vi "PH_Beckhoff_PP_PU.ProcPeriodic.vi"(0 "i ref in":refnum<vi>, 3 "ms timeout (10000)":i32=10000, 5 "error in (no error)":errorcluster) -> (14 "i ref out":refnum<vi>, 17 "timed out":bool, 19 "error out":errorcluster)   [LabVIEW 2014, in "PH_Beckhoff_PP_PU.lvlib"]
doc: "This method serves to periodically do things like reading values from the HW. Methods that should be executed periodically should be called from THIS methode. Add code here."
uses:
  PH_Beckhoff_PP_PU.lvlib
  PH_Beckhoff/PH_Beckhoff.lvlib
  non_GPL/instr.lib/Beckhoff/Beckhoff - Driver np.lvlib
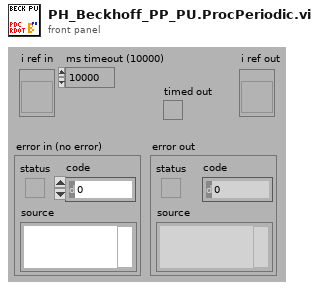
[diagram p1: front panel]
types:
  T1 = typedef "PH_Beckhoff_PP_PU.lvlib/PH_Beckhoff_PP_PU.i attribute.ctl" = cluster{"HV Meas":cluster{"Input GUI Ref":refnum<vi>, "Voltage Service ID":i32, "Voltage [V]":dbl, "Quality":bool, "# in Data":i32}[], "Trigger":cluster{"Status":cluster{"GUI Ref":refnum<vi>, "Status Service ID":i32, "Status":T2}, "last shot:":cluster{"GUI Ref":refnum<vi>, "Service ID":i32, "Time":string}, "DIs":cluster{"triggered":cluster{"GUI Ref":refnum<vi>, "# in Data":i32}, "fired":cluster{"GUI Ref":refnum<vi>, "# in Data":i32}}, "GUI Ref Indicator":refnum<vi>}[], "RR":cluster{"Status":cluster{"GUI Ref":refnum<vi>, "Status Service ID":i32, "Status":T2}, "DIs":cluster{"closed":cluster{"GUI Ref":refnum<vi>, "# in Data":i32}, "open":cluster{"GUI Ref":refnum<vi>, "# in Data":i32}}, "Close":cluster{"GUI Ref":refnum<vi>, "# in Data":i32}, "GUI Ref Indicator":refnum<vi>}[], "Igni":cluster{"Status":cluster{"GUI Ref":refnum<vi>, "Status Service ID":i32, "Status":T2}, "DIs":cluster{"heating on":cluster{"GUI Ref":refnum<vi>, "# in Data":i32}, "water on":cluster{"GUI Ref":refnum<vi>, "# in Data":i32}}, "Device on":cluster{"GUI Ref":refnum<vi>, "# in Data":i32}, "GUI Ref Indicator":refnum<vi>}[], "PSU":cluster{"Status":cluster{"GUI Ref":refnum<vi>, "Status Service ID":i32, "Status":T2}, "Limit Service ID":i32, "DIs":cluster{"inhibit":cluster{"GUI Ref":refnum<vi>, "# in Data":i32}, "end of charge":cluster{"GUI Ref":refnum<vi>, "# in Data":i32}, "HV on":cluster{"GUI Ref":refnum<vi>, "# in Data":i32}, "overtemp":cluster{"GUI Ref":refnum<vi>, "# in Data":i32}, "interlock":cluster{"GUI Ref":refnum<vi>, "# in Data":i32}, "load fault":cluster{"GUI Ref":refnum<vi>, "# in Data":i32}, "sum fault":cluster{"GUI Ref":refnum<vi>, "# in Data":i32}, "HV off":cluster{"GUI Ref":refnum<vi>, "# in Data":i32}, "DC ok":cluster{"GUI Ref":refnum<vi>, "# in Data":i32}}, "AIs":cluster{"voltage":cluster{"GUI Ref":refnum<vi>, "# in Data":i32}, "current":cluster{"GUI Ref":refnum<vi>, "# in Data":i32}}, "DAs":cluster{"inhibit":cluster{"GUI Ref":refnum<vi>, "# in Data":i32}, "interlock":cluster{"GUI Ref":refnum<vi>, "# in Data":i32}, "HV on":cluster{"GUI Ref":refnum<vi>, "# in Data":i32}, "Reset":cluster{"GUI Ref":refnum<vi>, "# in Data":i32}}, "AAs":cluster{"Voltage to set":cluster{"GUI Ref":refnum<vi>, "# in Data":i32}}, "GUI Ref Indicator":refnum<vi>}[], "reconfigured":cluster{"?":bool, "GUI Ref":refnum<vi>}, "PU Rack Type":T3, "HV Meas Info":T4, "PSU Info":T5}
  T2 = typedef "PH_StatusHandler.lvlib/PH_StatusHandler.Status.ctl" = i16
  T3 = typedef "PH_Beckhoff_PP_PU.lvlib/PH_Beckhoff_PP_PU.PU Rack Type.ctl" = enum16{"no Info", "PA 19mm", "PA 45mm", "MA PU 1 and 2", "MA PU 3 and 4", "MA PU 5 and 6", "MA FR and PILC"}
  T4 = typedef "PH_Beckhoff_PP_PU.lvlib/PH_Beckhoff_PP_PU.HV Meas Info.ctl" = cluster{"Period Time [s]":dbl, "Subtractor 1 [Hz]":dbl, "Devider 1 [Hz/kV]":dbl, "Subtractor 2 [Hz]":dbl, "Devider 2 [Hz/kV]":dbl}
  T5 = typedef "PH_Beckhoff_PP_PU.lvlib/PH_Beckhoff_PP_PU.PSU Info.ctl" = cluster{"Limits 1 [V]":cluster{"Lower":dbl, "Upper":dbl}, "Limits 2 [V]":cluster{"Lower":dbl, "Upper":dbl}}
  T6 = typedef "PH_Beckhoff.lvlib/PH_Beckhoff.i attribute.ctl" = cluster{"GUI Refs":T7, "operation?":bool, "Default Prdc Interval":i32, "Connection":T8, "AMS Net ID":T9, "Klemmencluster: # of":T10, "Values":T11, "IP":string, "Description":string, "configured?":bool, "Change Manager":cluster{"Detemination wanted?":bool, "Values changed at":cluster{"Sonderklemmen Inputs":i32[], "Analog Inputs":i32[], "Analog Outputs":i32[], "Digital Inputs":i32[], "Digital Outputs":i32[]}}, "Difference to handle an analog input as change":u32}
  T7 = typedef "PH_Beckhoff.lvlib/PH_Beckhoff.GUI Refs.ctl" = cluster{"ADS Error":refnum<vi>, "Values":refnum<vi>, "configured?":refnum<vi>, "Connection":refnum<vi>, "IP":refnum<vi>, "Prdc Int [ms]":refnum<vi>}
  T8 = typedef "PH_Beckhoff.lvlib/PH_Beckhoff.Connectivity.ctl" = cluster{"DLL?":bool, "Port?":bool, "Client?":bool, "Ping?":bool, "unsuccessful Pings":u32}
  T9 = typedef "Beckhoff - Driver np.lvlib/Beckhoff Access.ctl" = cluster{"DLL path":path, "AMS Net ID":cluster{"1st # of IP":u8, "2nd # of IP":u8, "3rd # of IP":u8, "4th # of IP":u8, "In Port":u8, "Out Port":u8}}
  T10 = typedef "Beckhoff - Driver np.lvlib/Klemmendeclarer.ctl" = cluster{"Offset due to Sonderklemms":u32, "analog Inputs":u32, "analog Outputs":u32, "digital Input Bits":u32, "digital Output Bits":u32}
  T11 = typedef "PH_Beckhoff.lvlib/PH_Beckhoff.Values.ctl" = cluster{"Sonderklemmen Inputs":T12, "Analog Inputs":T13, "Analog Outputs":T15, "Digital Inputs":T16, "Digital Outputs":T17}
  T12 = typedef "PH_Beckhoff.lvlib/PH_Beckhoff.Sonderklemmen Inputs.ctl" = cluster{"Total Length":u32, "Name":string, "Value":u64, "Quality":bool, "Service ID":i32, "Offset":u32, "Length":u32}[]
  T13 = typedef "PH_Beckhoff.lvlib/PH_Beckhoff.Analog Inputs.ctl" = cluster{"Name":string, "Value":u32, "Quality":bool, "Service ID":i32, "Sca Type":T14}[]
  T14 = typedef "PH_Beckhoff.lvlib/PH_Beckhoff.Scaling Type.ctl" = enum16{"none", "0 ... 15 Bit -> 0 ... 5", "0 ... 15 Bit -> 0 ... 10", "0 ... 15 Bit -> 0 ... 25", "0 ... 15 Bit -> 4 ... 20", "0 ... 15 Bit -> 0 ... 1", "0 ... 15 Bit -> 0 ... 20000", "0 ... 15 Bit -> 0 ... 24000"}
  T15 = typedef "PH_Beckhoff.lvlib/PH_Beckhoff.Analog Outputs.ctl" = cluster{"Name":string, "Value":u32, "Quality":bool, "Wanted Value":u32, "Service ID":i32, "Sca Type":T14}[]
  T16 = typedef "PH_Beckhoff.lvlib/PH_Beckhoff.Digital Inputs.ctl" = cluster{"Name":string, "Value":bool, "Quality":bool, "Service ID":i32, "inverted?":bool}[]
  T17 = typedef "PH_Beckhoff.lvlib/PH_Beckhoff.Digital Outputs.ctl" = cluster{"Name":string, "Value":bool, "Quality":bool, "Wanted Value":bool, "Service ID":i32, "inverted?":bool}[]
  T18 = cluster{"Sonderklemmen Inputs":i32[], "Analog Inputs":i32[], "Analog Outputs":i32[], "Digital Inputs":i32[], "Digital Outputs":i32[]}
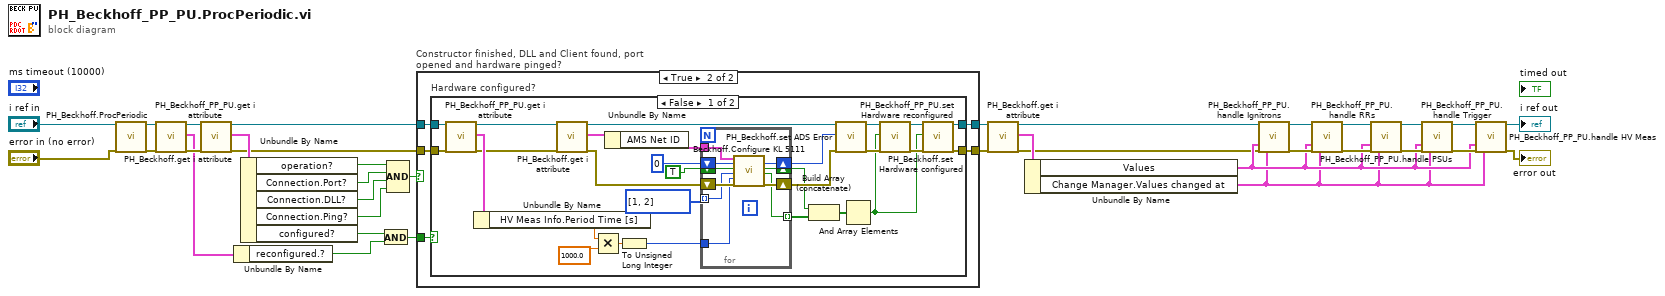
[diagram p0: block diagram]
diagram:
  n1 = call "PH_Beckhoff.ProcPeriodic.vi"("i ref in"="i ref in", "error in (no error)"="error in (no error)") -> ("i ref out"=w6:refnum<vi>, "error out"=w27:errorcluster)  [unwired: 15 in, 1 out]
  n2 = call "PH_Beckhoff_PP_PU.get i attribute.vi"("i ref in"=w6, "error in (no error)"=w27) -> ("i ref out"=w5:refnum<vi>, "i attribute"=w4:T1, "error out"=w7:errorcluster)  [unwired: 15 in]
  n3 = call "PH_Beckhoff.get i attribute.vi"("i ref in"=w5, "error in (no error)"=w7) -> ("i ref out"=w31:refnum<vi>, "i attribute"=w33:T6, "error out"=w30:errorcluster)  [unwired: 15 in]
  n4 = Unbundle By Name(w4) -> ("reconfigured.?"=w3:bool)
  n5 = Unbundle By Name(w33) -> ("operation?"=w21:bool, "Connection.Port?"=w29:bool, "Connection.DLL?"=w28:bool, "Connection.Ping?"=w20:bool, "configured?"=w2:bool)
  n6 = And(x=w2, y=w3) -> (x .and. y?=w1:bool)
  n7 = Compound Arithmetic op=AND(w21, w29, w28, w20) -> (w32:bool)
  n8 = case "Constructor finished, DLL and Client found, port opened and hardware pinged?" shown="True" w32 {
    tunnel: w30 -> [w36 w41]
    tunnel: w31 -> [w37 w42]
    tunnel: [w36 w39] -> w22
    tunnel: [w37 w40] -> w23
    tunnel: w1 -> [_ w38]
    frame False {
    }
    frame True {
      n9 = case "Hardware configured?" shown="False" w38 {
        tunnel: [w45 w82] -> w40
        tunnel: [w44 w81] -> w39
        tunnel: w41 -> [w69 w81]
        tunnel: w42 -> [w70 w82]
        frame False {
          n10 = call "PH_Beckhoff_PP_PU.get i attribute.vi"("i ref in"=w70, "error in (no error)"=w69) -> ("i ref out"=w52:refnum<vi>, "i attribute"=w68:T1, "error out"=w51:errorcluster)  [unwired: 15 in]
          n11 = Unbundle By Name(w68) -> ("HV Meas Info.Period Time [s]"=w48:dbl)
          n12 = call "PH_Beckhoff.get i attribute.vi"("i ref in"=w52, "error in (no error)"=w51) -> ("i ref out"=w61:refnum<vi>, "i attribute"=w54:T6, "error out"=w57:errorcluster)  [unwired: 15 in]
          n13 = Multiply(x=w48, y=1000.0) -> (x*y=w66:dbl)
          n14 = Unbundle By Name(w54) -> ("AMS Net ID"=w55:T9)
          n15 = To Unsigned Long Integer(number=w66) -> (unsigned 32bit integer=w53:u32)
          n16 = for {
            tunnel: w55 -> [w79]
            tunnel: w53 -> [w77]
            shift-right: [w76] -> w63
            shift-left: w57 -> [w80]
            shift-right: [w75] -> w58
            shift-left: TRUE ("Do it?") -> [w78]
            tunnel: [w74] -> w59 mode=indexing
            tunnel: u32[] [1, 2] -> [w73] mode=indexing
            shift-right: [w71] -> w50
            shift-left: 0 ("ADS Error out") -> [w72]
            n17 = call "Beckhoff.Configure KL 5111.vi"("AMS Net ID in"=w79, "ADS Error in (0)"=w72, "Do it?"=w78, "# to configure"=w73, "Timewindow [ms]"=w77, "error in"=w80) -> ("ADS Error out"=w71:i32, "Process successful?"=w75:bool, "KL 5111 configured?"=w74:bool, "error out"=w76:errorcluster)  [unwired: 8 in, 2 out]
          }
          n18 = Build Array (concatenate)(w58, w59) -> (w60:bool[])
          n19 = call "PH_Beckhoff.set ADS Error.vi"("i ref in"=w61, "ADS Error"=w50, "error in"=w63) -> ("i ref out"=w62:refnum<vi>, "error out"=w64:errorcluster)  [unwired: 15 in]
          n20 = And Array Elements(Boolean array=w60) -> (logical AND=w43:bool)
          n21 = call "PH_Beckhoff.set Hardware configured.vi"("i ref in"=w62, "Hardware configured?"=w43, "error in"=w64) -> ("i ref out"=w46:refnum<vi>, "error out"=w47:errorcluster)  [unwired: 15 in]
          n22 = call "PH_Beckhoff_PP_PU.set Hardware reconfigured.vi"("i ref in"=w46, "Hardware reconfigured?"=w43, "error in"=w47) -> ("i ref out"=w45:refnum<vi>, "error out"=w44:errorcluster)  [unwired: 15 in]
        }
        frame True {
        }
      }
    }
  }
  n23 = call "PH_Beckhoff.get i attribute.vi"("i ref in"=w23, "error in (no error)"=w22) -> ("i ref out"=w9:refnum<vi>, "i attribute"=w24:T6, "error out"=w8:errorcluster)  [unwired: 15 in]
  n24 = Unbundle By Name(w24) -> ("Values"=w11:T11, "Change Manager.Values changed at"=w10:T18)
  n25 = call "PH_Beckhoff_PP_PU.handle Ignitrons.vi"("i ref in"=w9, "Values"=w11, "error in"=w8, "Values changed at"=w10) -> ("i ref out"=w18:refnum<vi>, "error out"=w16:errorcluster)  [unwired: 14 in]
  n26 = call "PH_Beckhoff_PP_PU.handle RRs.vi"("i ref in"=w18, "Values"=w11, "error in"=w16, "Values changed at"=w10) -> ("i ref out"=w17:refnum<vi>, "error out"=w15:errorcluster)  [unwired: 14 in]
  n27 = call "PH_Beckhoff_PP_PU.handle PSUs.vi"("i ref in"=w17, "Values"=w11, "error in"=w15, "Values changed at"=w10) -> ("i ref out"=w13:refnum<vi>, "error out"=w19:errorcluster)  [unwired: 14 in]
  n28 = call "PH_Beckhoff_PP_PU.handle Trigger.vi"("i ref in"=w13, "Values"=w11, "error in"=w19, "Values changed at"=w10) -> ("i ref out"=w12:refnum<vi>, "error out"=w14:errorcluster)  [unwired: 14 in]
  n29 = call "PH_Beckhoff_PP_PU.handle HV Meas.vi"("i ref in"=w12, "Values"=w11, "error in"=w14, "Values changed at"=w10) -> ("i ref out"=→"i ref out":refnum<vi>, "error out"=→"error out":errorcluster)  [unwired: 14 in]
